vi "MainNR.vi"(10 "JQMHStartup":refnum<class "JQMHStartup.lvclass">, 11 "TesterModule in":refnum<class "TesterModule.lvclass">) -> ()   [LabVIEW 2024, in "TesterModule.lvclass"]
uses:
  TesterModule.lvclass
  C:/Github/JQMH/JQMHCore/Module/JQMHModule.lvclass
  JQMHCore/JQMHStartup/JQMHStartup.lvclass
  JQMHCore/Module/JQMHModule.lvclass/JQMHModule.ctl
  TesterModule.lvclass/TesterModule.ctl
  Message Queue_class/RQMHMessageQueue.lvclass/RQMHMessageQueue.ctl
  Message Queue_class/Delacor_lib_QMH_Enqueue Message (Single).vi
  Message Queue_class/RQMHMessageQueue.lvclass
  JQMHCore/Module/JQMHModule.lvclass
  C:/Github/JQMH/TesterModule/TesterModule.lvclass
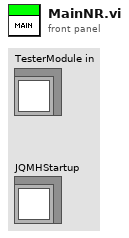
[diagram p1: front panel]
types:
  T1 = typedef "TesterModule.lvclass/Request Events--cluster.ctl" = cluster{"NewControl78732508":refnum<user-event>, "Load Big Data":refnum<user-event>}
  T2 = typedef "JQMHModule.lvclass/StandardRequests.ctl" = cluster{"Initialise":refnum<user-event>, "Stop Module":refnum<user-event>, "ShowFP":refnum<user-event>, "Hide Front Panel":refnum<user-event>, "Show Block Diagram":refnum<user-event>, "Hide Block Diagram":refnum<user-event>}
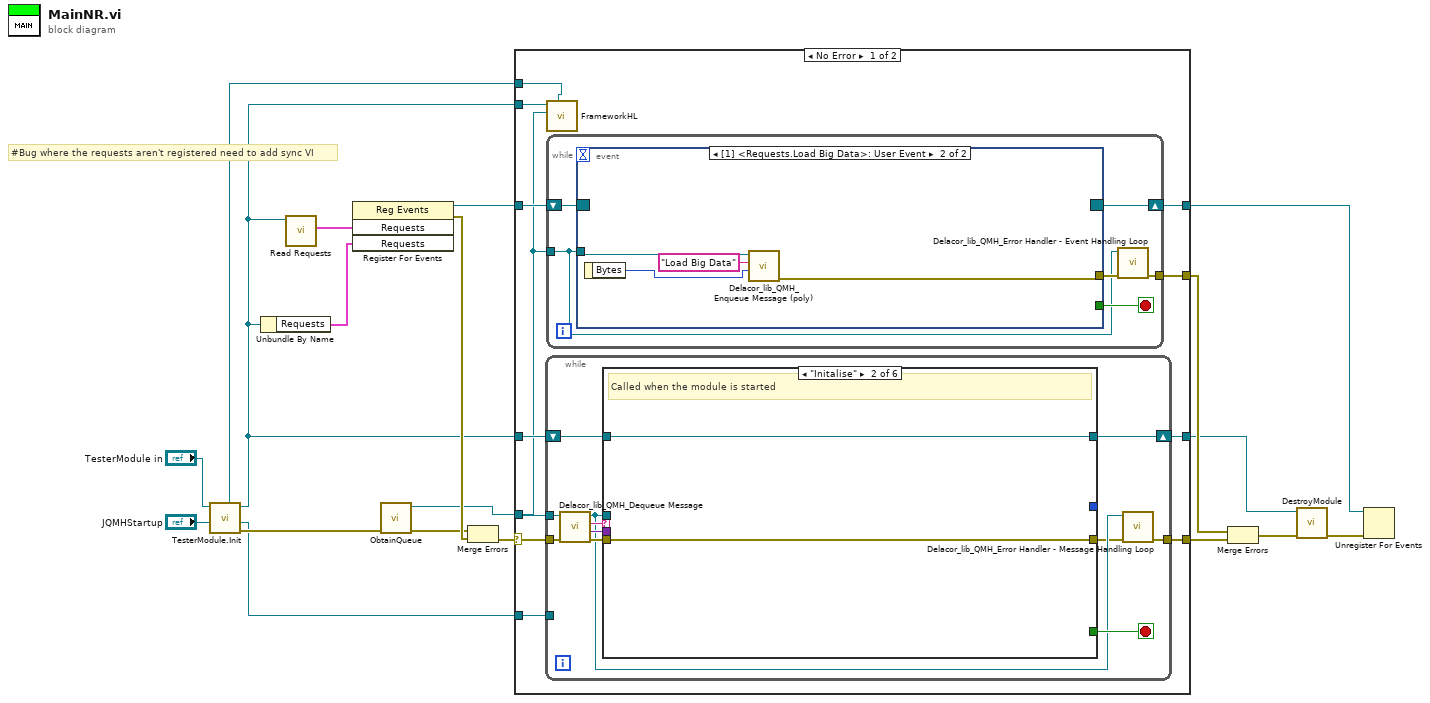
[diagram p0: block diagram]
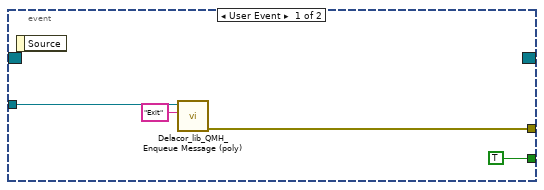
[diagram p2: hidden frame]
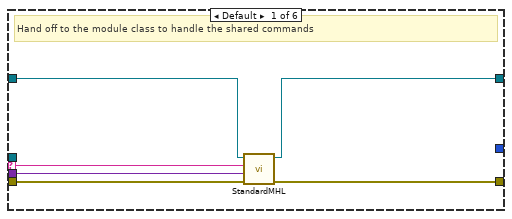
[diagram p3: hidden frame]
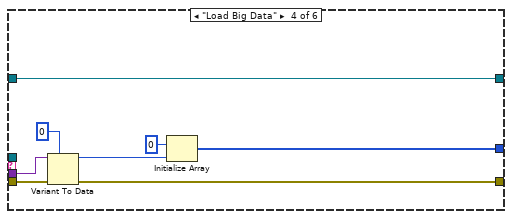
[diagram p5: hidden frame]
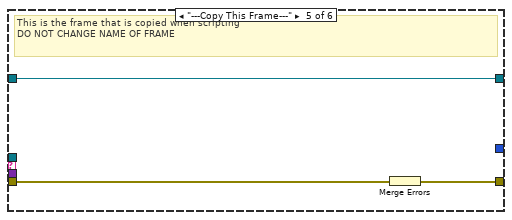
[diagram p6: hidden frame]
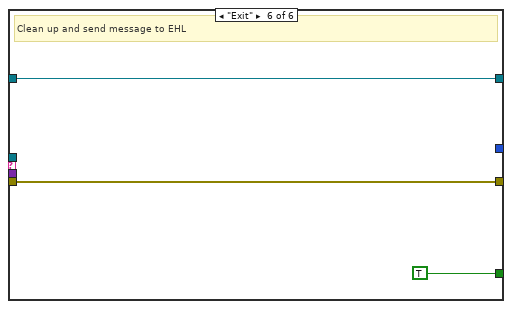
[diagram p7: hidden frame]
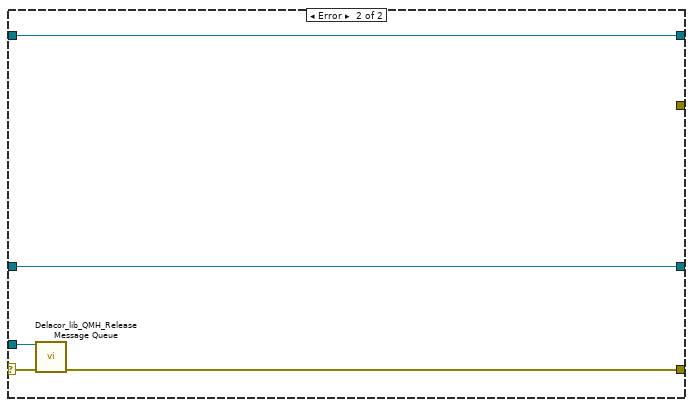
[diagram p8: hidden frame]
diagram:
  # "#Bug where the requests aren't registered need to add sync VI"
  n1 = call "TesterModule.Init.vi"("JQMHStartup in"="JQMHStartup", "TesterModule in"="TesterModule in") -> ("error out"=w5:errorcluster, "JQMHStartup out"=w2:refnum<class "JQMHStartup.lvclass">, "TesterModule out"=w4:refnum<class "TesterModule.lvclass">, "Event Registration Refnum"=w1:refnum<event-registration>)  [unwired: 4 in, 2 out]
  n2 = Unbundle By Name(w4) -> ("Requests"=w7:T1)
  n3 = call "Read Requests.vi"("JQMHModule in"=w4) -> ("Requests"=w6:T2)  [unwired: 9 in, 1 out]
  n4 = register-events(w6, w7) -> (reference out=w17:refnum<event-registration>, error out=w19:errorcluster)  [unwired: 2 in]
  n5 = call "ObtainQueue.vi"("error in"=w5) -> ("error out"=w15:errorcluster, "Message Queue"=w16:refnum<class "RQMHMessageQueue.lvclass">)  [unwired: 9 in]
  n6 = Merge Errors(w15, w19) -> (w13:errorcluster)
  n7 = case "JQMH_Main" shown="No Error" w13 {
    selector: w13 -> [w26 w82]
    tunnel: w4 -> [w30 w80]
    tunnel: [w29 w84] -> w18
    tunnel: w17 -> [w28 w84]
    tunnel: w16 -> [w21 w83]
    tunnel: [w27 w81] -> w14
    tunnel: [w25 _] -> w12
    tunnel: [w24 w80] -> w9
    tunnel: w4 -> [w23 _]
    tunnel: w2 -> [w22 _]
    tunnel: w1 -> [w20 _]
    frame No Error {
      n8 = while {
        tunnel: w21 -> [w55]
        tunnel: w26 -> [w53]
        shift-right: [w46] -> w24
        shift-left: w30 -> [w51]
        tunnel: [w45] -> w27
        tunnel: w22 -> [_]
        stop <- w52 stop-if-true
        n9 = call-dynamic "Delacor_lib_QMH_Dequeue Message.vi"("error in"=w53, "Message Queue in"=w55) -> ("error out"=w49:errorcluster, "Message Data"=w50:variant, "Message"=w54:string, "Message Queue out"=w48:refnum<class "RQMHMessageQueue.lvclass">)  [unwired: 6 in]
        n10 = case "JQMH_MESSAGE_CASES" shown="\"Initalise\"" w54 {
          selector: w54 -> [w58 _ _ _ _ _]
          tunnel: [_ _ _ _ _ TRUE] -> w52
          tunnel: w51 -> [w59 w63 w64 w73 w75 w77]
          tunnel: w50 -> [w57 _ _ w70 _ _]
          tunnel: w49 -> [w60 w62 w65 w71 w76 w78]
          tunnel: w48 -> [_ _ _ _ _ _]
          tunnel: [w61 w62 w65 w72 w74 w78] -> w47
          tunnel: [w56 w63 w64 w73 w75 w77] -> w46
          tunnel: [_ _ _ w66 _ _] -> _
          frame Default {
            # "Hand off to the module class to handle the shared commands"
            n11 = call-dynamic "StandardMHL.vi"("error in (no error)"=w60, "Message Data"=w57, "Message"=w58, "JQMHModule in"=w59) -> ("error out"=w61:errorcluster, "JQMHModule out"=w56:refnum<class "TesterModule.lvclass">)  [unwired: 6 in]
          }
          frame "Initalise" {
            # "Called when the module is started"
          }
          frame "---Module Specific---" {
          }
          frame "Load Big Data" {
            n12 = Variant To Data(error in=w71, type=u32 0 ("element"), Variant=w70) -> (data=w68:u32, error out=w72:errorcluster)
            n13 = Initialize Array(u8 0 ("element"), w68) -> (w66:u8[])
          }
          frame "---Copy This Frame---" {
            # "This is the frame that is copied when scripting\nDO NOT CHANGE NAME OF FRAME"
            n14 = Merge Errors(w76) -> (w74:errorcluster)
          }
          frame "Exit" {
            # "Clean up and send message to EHL"
          }
        }
        n15 = call-dynamic "Delacor_lib_QMH_Error Handler - Message Handling Loop.vi"("error in"=w47, "Message Queue in"=w48) -> ("dup error in"=w45:errorcluster)  [unwired: 8 in, 1 out]
      }
      n16 = call-dynamic "FrameworkHL.vi"("StandardRequests"=w20, "Message Queue"=w21, "JQMHModule in"=w23) -> ()  [unwired: 9 in]
      n17 = while {
        shift-right: [w35] -> w29
        shift-left: w28 -> [w36]
        tunnel: w21 -> [w31]
        tunnel: [w32] -> w25
        stop <- w34 stop-if-true
        n18 = event "JQMH_EVENT_MAIN" shown="[1] <Requests.Load Big Data>: User Event" {
          selector: w36 -> [_ _]
          dyn-events: [_ _] -> w35
          timeout: _ -> [_ _]
          tunnel: [TRUE _] -> w34
          tunnel: w31 -> [w39 w44]
          tunnel: [w37 w41] -> w33
          event User Event {
            n19 = event-data() -> ()  [unwired: 1 in, 1 out]
            n20 = call-poly "Delacor_lib_QMH_Enqueue Message (poly).vi"("Message"="Exit", "Message Queue in"=w39) -> ("error out"=w37:errorcluster)  [unwired: 8 in, 1 out]
          }
          event User Event {
            n21 = event-data() -> ("Bytes"=w42:u32)  [unwired: 1 in]
            n22 = call-poly "Delacor_lib_QMH_Enqueue Message (poly).vi"("Message Data"=w42, "Message"="Load Big Data", "Message Queue in"=w44) -> ("error out"=w41:errorcluster)  [unwired: 7 in, 1 out]
          }
        }
        n23 = call-dynamic "Delacor_lib_QMH_Error Handler - Event Handling Loop.vi"("error in"=w33, "Message Queue in"=w31) -> ("dup error in"=w32:errorcluster)  [unwired: 8 in, 1 out]
      }
    }
    frame Error {
      n24 = call-dynamic "Delacor_lib_QMH_Release Message Queue.vi"("error in"=w82, "Message Queue"=w83) -> ("error out"=w81:errorcluster)  [unwired: 9 in]
    }
  }
  n25 = Merge Errors(w12, w14) -> (w11:errorcluster)
  n26 = call "DestroyModule.vi"("error in (no error)"=w11, "JQMHModule in"=w9) -> ("error out"=w10:errorcluster)  [unwired: 9 in]
  n27 = Unregister For Events(event registration refnum=w18, error in=w10) -> ()  [unwired: 1 out]
